vi "Submit Order.vi"(8 "error in (no error)":errorcluster, 10 "Order Content":cluster{"Drink type":T1, "Options":T2[]}[](array[cluster]), 11 "Customer In":refnum<class "Customer.lvclass">) -> (0 "error out":errorcluster, 3 "Customer Out":refnum<class "Customer.lvclass">)   [LabVIEW 2020, in "Customer.lvclass"]
uses:
  Customer.lvclass
  C:/Program Files (x86)/National Instruments/LabVIEW 2020/vi.lib/Asteme/Triarc Framework/Process/Process.lvclass
  Support/Beverages/TypeDefs/Drink Type.ctl
  Support/Beverages/TypeDefs/Options.ctl
  <vilib>/Asteme/Triarc Framework/Process/Process.lvclass/Process.ctl
  <vilib>/AdvancedString/1D String Array to Delimited String.vi
  <vilib>/Asteme/Triarc Framework/Process/Public/Lifecycle/Get Lifecycle State.vi
  <vilib>/Utility/error.llb/Clear Errors.vi
  <vilib>/Utility/error.llb/Error Cluster From Error Code.vi
  <vilib>/Asteme/Triarc Framework/Process/Process.lvclass
  Support/Beverages/Beverage/Beverage.lvclass
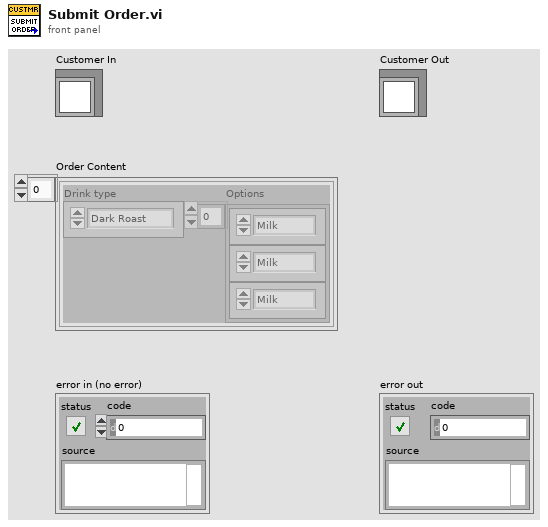
[diagram p1: front panel]
types:
  T1 = typedef "Beverage.lvclass/Drink Type.ctl" = enum16{"Dark Roast", "Decaf", "Espresso", "House Blend"}
  T2 = typedef "Beverage.lvclass/Options.ctl" = enum16{"<None>", "Milk", "Mocha", "Soy", "Whip"}
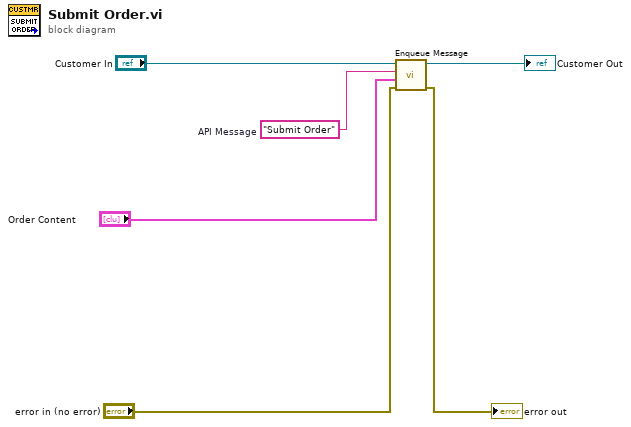
[diagram p0: block diagram]
diagram:
  w3 = "Submit Order"  # API Message
  n1 = call <vilib>:"Enqueue Message.vi"("error in (no error)"="error in (no error)", "Message Data"="Order Content", "Message"=w3, "Process In"="Customer In") -> ("error out"=→"error out":errorcluster, "Process Out"=→"Customer Out":refnum<class "Customer.lvclass">)  [unwired: 6 in]
